vi "Camera_AcquireSingleImage.vi"(2 "error in":errorcluster) -> (0 "error out":errorcluster, 1 "Image Out":T1(plugin-control))   [LabVIEW 2009, in "Camera.lvlib"]
uses:
  Camera.lvlib
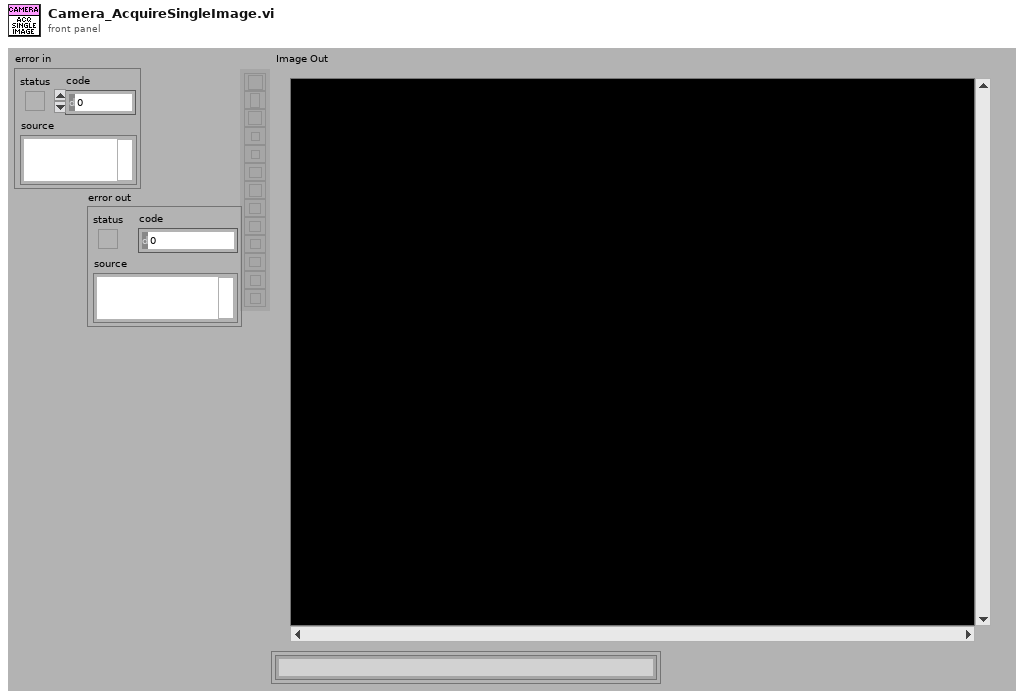
[diagram p1: front panel]
types:
  T1 = typedef "IMAQ Image.ctl" = refnum<image>
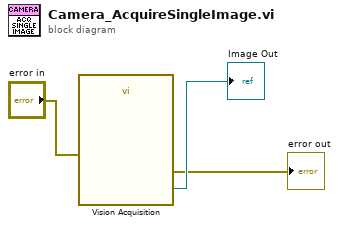
[diagram p0: block diagram]
diagram:
  n1 = call "Vision Acquisition"("error in"="error in") -> ("Image Out"=→"Image Out":T1, "error out"=→"error out":errorcluster)  [unwired: 25 in]
